vi "Latch Timeout.vi"(9 "Timeout?":bool, 10 "Clear":bool) -> (1 "Ever Timed Out?":bool)   [LabVIEW 2012]
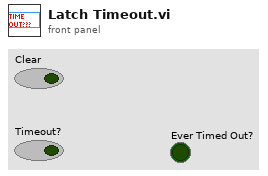
[diagram p1: front panel]
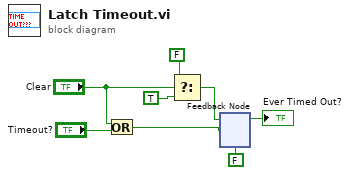
[diagram p0: block diagram]
diagram:
  n1 = Or(x="Clear", y="Timeout?") -> (x .or. y?=w5:bool)
  n2 = Select(t=FALSE, s="Clear", f=TRUE) -> (s? t:f=w1:bool)
  n3 = feedback #1(FALSE) -> (→"Ever Timed Out?":bool)
  n4 = feedback-in #1(w1, w5) -> ()
